vi "Set Request Queue.vi"(8 "error in (no error)":errorcluster, 10 "request_queue":refnum<queue>, 11 "output_poller_queue in":refnum<class "output_poller_queue.lvclass">) -> (0 "error out":errorcluster, 3 "output_poller_queue out":refnum<class "output_poller_queue.lvclass">)   [LabVIEW 2015, in "output_poller_queue.lvclass"]
uses:
  output_poller_queue.lvclass
  request/request.lvclass
  output_poller_queue.lvclass/output_poller_queue.ctl
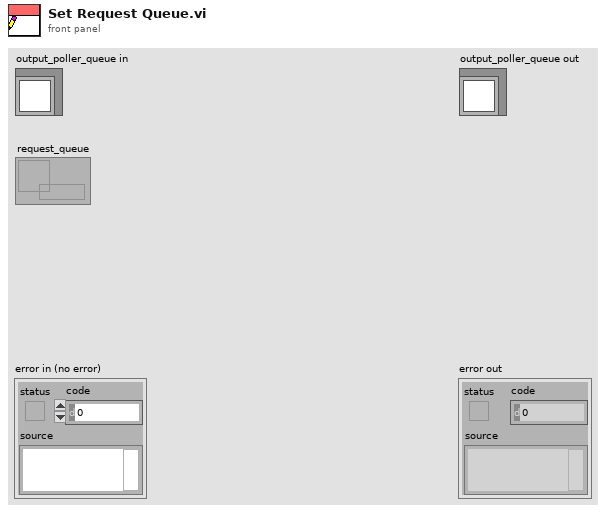
[diagram p1: front panel]
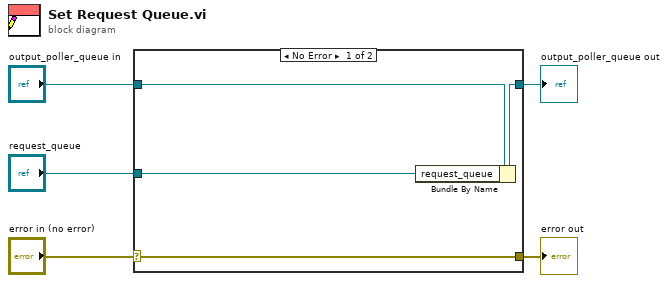
[diagram p0: block diagram]
diagram:
  n1 = case shown="No Error" "error in (no error)" {
    selector: "error in (no error)" -> [w9 w10]
    tunnel: [w9 w10] -> w4
    tunnel: [w7 w11] -> w2
    tunnel: "output_poller_queue in" -> [w8 w11]
    tunnel: "request_queue" -> [w6 _]
    frame No Error {
      n2 = Bundle By Name(cluster=w8, "request_queue"=w6) -> (w7:refnum<class "output_poller_queue.lvclass">)
    }
    frame Error {
    }
  }
  "error out" <- w4
  "output_poller_queue out" <- w2
